vi "Entry.vi"(8 "error in (no error)":errorcluster, 11 "New State":refnum<class "Manual.lvclass">) -> (0 "error out":errorcluster, 3 "State out":refnum<class "Manual.lvclass">)   [LabVIEW 2014, in "States.lvlib" / "Manual.lvclass"]
doc: "This is an abstract method. Override this method to define the behavior when you enter the state."
uses:
  Manual.lvclass
  ctl/P3AT_Current.ctl
  Global_var/Global_var.vi
  Process State/CoordinatorState.lvclass
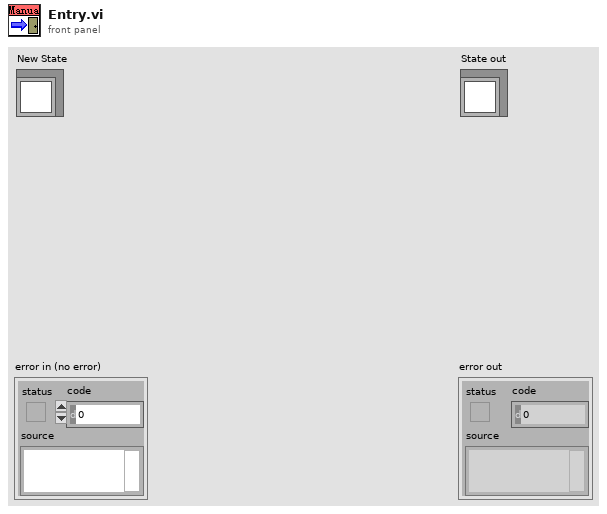
[diagram p1: front panel]
types:
  T1 = enum32{"Joy", "Map", "Voice", "Input", "Undefined"}
  T2 = typedef "P3AT_Current.ctl" = cluster{"max_vel":dbl, "max_rot":dbl, "now_pose_X":dbl, "now_pose_Y":dbl, "now_pose_Rot_deg":dbl, "Control_Mode":enum32{"Joy", "Map", "Voice", "Input", "Undefined"}}
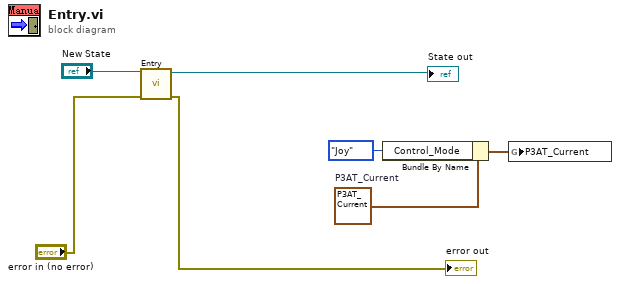
[diagram p0: block diagram]
diagram:
  w3 = T2 {"max_vel"=0.49056603773584906, "max_rot"=0.5094339622641509, "now_pose_X"=0.0, "now_pose_Y"=0.0, "now_pose_Rot_deg"=0.0, "Control_Mode"=enum."Joy"}  # P3AT_Current
  n1 = call-parent "Entry.vi"("error in (no error)"="error in (no error)", "New State"="New State") -> ("error out"=→"error out":errorcluster, "State out"=→"State out":refnum<class "Manual.lvclass">)  [unwired: 8 in]
  n2 = Bundle By Name(cluster=w3, "Control_Mode"=T1."Joy") -> (w2:T2)
  n3 = global write "Global_var.vi" "P3AT_Current"(w2) -> ()
